vi "macro_Rotation3d_Axis_AngleDeg.vi"   [LabVIEW 2019, in "Trajectory_Library.lvlib"]
uses:
  Trajectory_Library.lvlib
  Matrix_NormF.vi
  VI/Quaternion_New.vi
  VI/Rotation3d_Create_Default.vi
  <vilib>/Analysis/_algsub.llb/Matrix Norm.vi
  <vilib>/Analysis/_algsub.llb/Real Matrix Norm.vi
  VI/Quaternion_New_Default.vi
  <vilib>/Analysis/Matrix/Numeric/Conversions/Array To Matrix.vi
  <vilib>/Analysis/Matrix/Numeric/Conversions/Array To Matrix - RA.vi
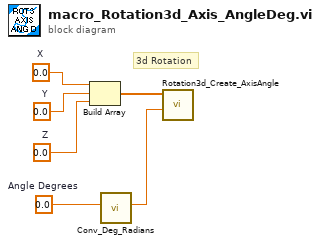
[diagram p0: block diagram]
diagram:
  w1 = 0.0  # Angle Degrees
  w3 = 0.0  # Z
  w5 = 0.0  # X
  w4 = 0.0  # Y
  # "3d Rotation"
  n1 = Build Array(w5, w4, w3) -> (w6:dbl[])
  n2 = call "Conv_Deg_Radians.vi"("Degress"=w1) -> ("Radians"=w2:dbl)  [unwired: 10 in]
  n3 = call "Rotation3d_Create_AxisAngle.vi"("Angle"=w2, "Axis Vector"=w6) -> ()  [unwired: 9 in, 1 out]
